vi "Version 1_Write Communication Settings.vi"(6 "Change Unit Data Rate (NOT USED)":T1(ring), 7 "Unit ID (A)":string="A", 8 "error in":errorcluster, 9 "Change Unit Baud Rate":enum8{"2400", "9600", "19200", "38400"}(ring)=enum."19200", 10 "Change Unit ID":string, 11 "VISA Session In":refnum<visa-resource-name>="Alicat") -> (0 "error out":errorcluster, 3 "VISA Session Out":refnum<visa-resource-name>)   [LabVIEW 2016]
doc: "Changes the baud rate or the unit ID of an Alicat device."
panel:
  # "Unused, since all 80000+\nserial numbers don't use \nthis feature"
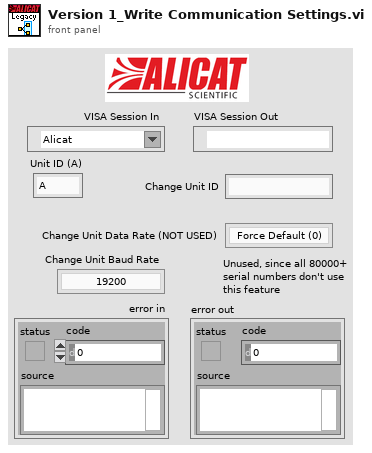
[diagram p1: front panel]
types:
  T1 = enum8{"Force Default (0)", "Fast (Char)", "Slow (IDLE+Char)", "Force Default (3)", "Unused"}
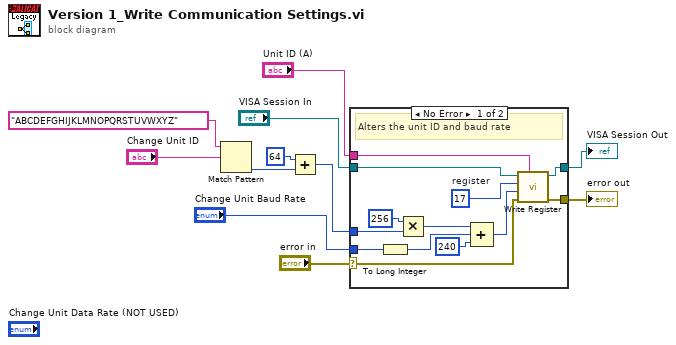
[diagram p0: block diagram]
diagram:
  n1 = Match Pattern(string="ABCDEFGHIJKLMNOPQRSTUVWXYZ", regular expression="Change Unit ID") -> (offset past match=w3:i32)  [unwired: 1 in, 3 out]
  n2 = Add(x=64, y=w3) -> (x+y=w1:i32)
  n3 = case shown="No Error" "error in" {
    selector: "error in" -> [w12 w26]
    tunnel: "VISA Session In" -> [w23 w25]
    tunnel: "Unit ID (A)" -> [w22 _]
    tunnel: [w21 w25] -> w9
    tunnel: [w20 w26] -> w8
    tunnel: "Change Unit Baud Rate" -> [w19 _]
    tunnel: w1 -> [w15 _]
    frame No Error {
      w24 = u16 17  # register
      # "Alters the unit ID and baud rate"
      n4 = To Long Integer(number=w19) -> (32bit integer=w18:i32)
      n5 = Multiply(x=256 ("y"), y=w15) -> (x*y=w14:i32)
      n6 = Compound Arithmetic op=ADD(w14, w18, 240 ("y")) -> (w16:i32)
      n7 = call "Write Register.vi"("Unit ID (A)"=w22, "error in"=w12, "Register Value"=w16, "Register address"=w24, "VISA Session In"=w23) -> ("error out"=w20:errorcluster, "VISA Session Out"=w21:refnum<visa-resource-name>)  [unwired: 4 in, 1 out]
    }
    frame Error {
    }
  }
  "error out" <- w8
  "VISA Session Out" <- w9
